vi "Set Pin Status.vi"(0 "Simulado in":refnum<class "Simulado.lvclass">, 5 "Port":dbl, 7 "Pin":dbl, 9 "Value":bool, 11 "error in (no error)":errorcluster) -> (4 "Simulado out":refnum<class "Simulado.lvclass">, 15 "error out":errorcluster)   [LabVIEW 2020, in "Simulado.lvclass"]
uses:
  Simulado.lvclass
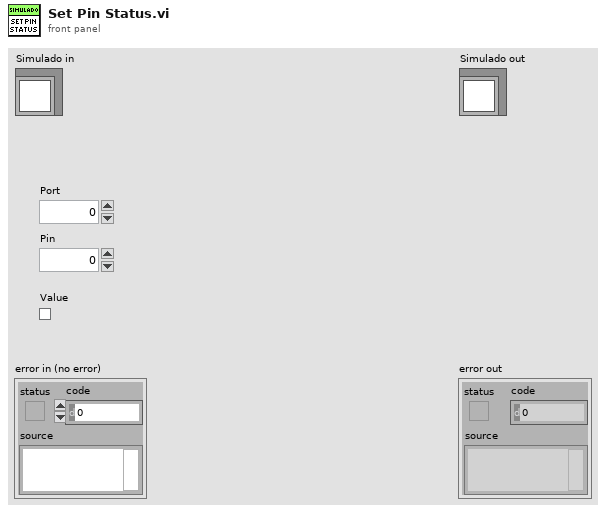
[diagram p1: front panel]
types:
  T1 = typedef "Serial device.lvclass/Brand combobox.ctl" = string
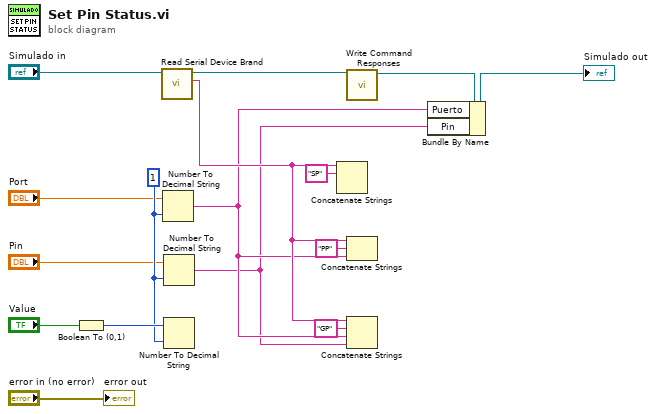
[diagram p0: block diagram]
diagram:
  w9 = i16 1 ("width (-)")
  n1 = Boolean To (0,1)(Boolean="Value") -> (0, 1=w11:i16)
  n2 = call-dynamic "Read Serial Device Brand.vi"("Serial device in"="Simulado in") -> ("Serial Device Brand"=w6:T1, "Serial device out"=w15:refnum<class "Simulado.lvclass">)  [unwired: 8 in, 1 out]
  n3 = Number To Decimal String(number="Port", width (-)=w9) -> (decimal integer string=w2:string)
  n4 = Number To Decimal String(number="Pin", width (-)=w9) -> (decimal integer string=w1:string)
  n5 = Number To Decimal String(number=w11, width (-)=w9) -> ()  [unwired: 1 out]
  n6 = Concatenate Strings(w6, "SP" ("string")) -> ()  [unwired: 2 in, 1 out]
  n7 = call-dynamic "Write Command Responses.vi"("Simulado in"=w15) -> ("Simulado out"=w14:refnum<class "Simulado.lvclass">)  [unwired: 9 in, 1 out]
  n8 = Concatenate Strings(w6, "PP" ("string"), w2) -> ()  [unwired: 1 out]
  n9 = Concatenate Strings(w6, "GP" ("string"), w2, w1) -> ()  [unwired: 1 out]
  n10 = Bundle By Name(cluster=w14, "Puerto"=w2, "Pin"=w1) -> (→"Simulado out":refnum<class "Simulado.lvclass">)
  "error out" <- "error in (no error)"
